vi "chaosui-crest-cu-setstate.vi"(5 "dev_state":T1=enum."init", 6 "timeout (10000)":i32=10000, 7 "cuname":string, 8 "handleConnection":T3) -> (0 "dev_error":bool, 1 "timestamp":u64, 2 "nok":i32, 3 "dev_state_out":T1, 4 "output out":string)   [LabVIEW 2014, in "chaosui-crest.lvlib"]
doc: "uint64_t chaos_crest_cu_get(chaos_crest_handle_t h,const char*cuname,char*output,int maxsize);"
uses:
  chaosui-crest.lvlib
  <vilib>/httpClient/ClientHandle.ctl
  ChaosDevState.ctl
  <vilib>/httpClient/LabVIEWHTTPClient.lvlib
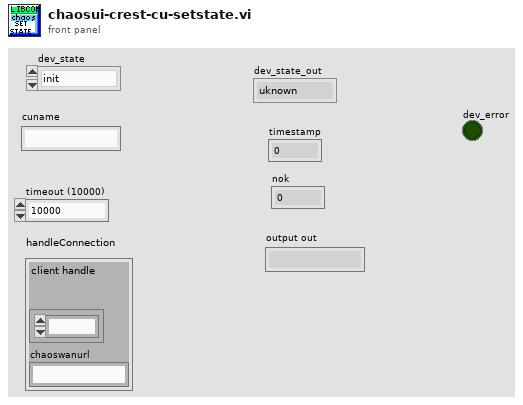
[diagram p1: front panel]
types:
  T1 = typedef "ChaosDevState.ctl" = enum16{"uknown", "stop", "init", "deinit", "start"}
  T2 = typedef "LabVIEWHTTPClient.lvlib/ClientHandle.ctl" = refnum<k1>
  T3 = cluster{"client handle":T2, "chaoswanurl":string}
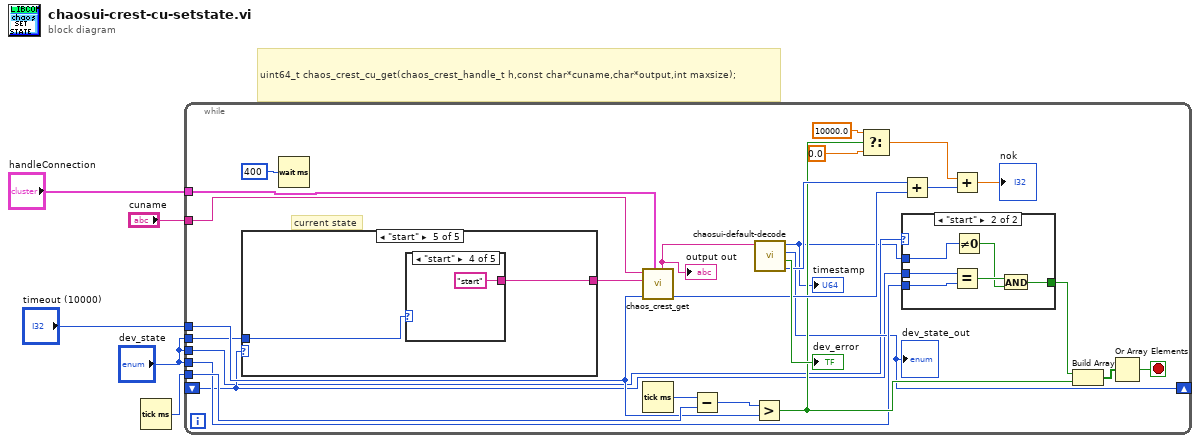
[diagram p0: block diagram]
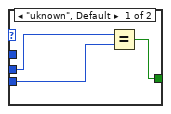
[diagram p2: hidden frame]
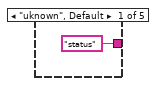
[diagram p3: hidden frame]
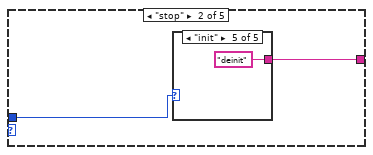
[diagram p4: hidden frame]
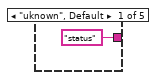
[diagram p5: hidden frame]
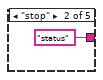
[diagram p6: hidden frame]
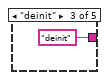
[diagram p7: hidden frame]
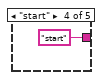
[diagram p8: hidden frame]
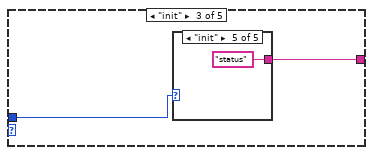
[diagram p9: hidden frame]
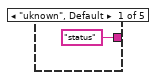
[diagram p10: hidden frame]
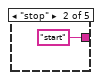
[diagram p11: hidden frame]
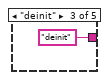
[diagram p12: hidden frame]
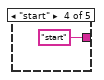
[diagram p13: hidden frame]
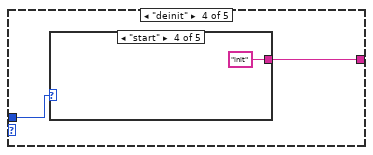
[diagram p14: hidden frame]
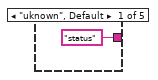
[diagram p15: hidden frame]
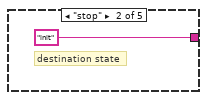
[diagram p16: hidden frame]
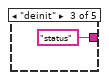
[diagram p17: hidden frame]
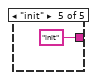
[diagram p18: hidden frame]
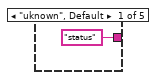
[diagram p19: hidden frame]
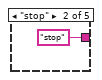
[diagram p20: hidden frame]
diagram:
  # "uint64_t chaos_crest_cu_get(chaos_crest_handle_t h,const char*cuname,char*output,int maxsize);"
  n1 = Tick Count (ms)() -> (millisecond timer value=w2:u32)
  n2 = while {
    tunnel: "handleConnection" -> [w30]
    tunnel: "timeout (10000)" -> [w21]
    tunnel: "cuname" -> [w29]
    tunnel: "dev_state" -> [w13]
    tunnel: w2 -> [w22]
    shift-right: [w11] -> _
    shift-left: _ -> [w10]
    tunnel: "dev_state" -> [w9]
    tunnel: "dev_state" -> [w8]
    stop <- w26 stop-if-true
    # "current state"
    n3 = case shown="\"start\"" w10 {
      tunnel: ["status" w43 w50 w57 w64] -> w12
      tunnel: w9 -> [_ w44 w51 w58 w65]
      frame "uknown", Default {
      }
      frame "stop" {
        n4 = case shown="\"init\"" w44 {
          tunnel: ["status" "status" "deinit" "start" "deinit"] -> w43
          frame "uknown", Default {
          }
          frame "stop" {
          }
          frame "deinit" {
          }
          frame "start" {
          }
          frame "init" {
          }
        }
      }
      frame "init" {
        n5 = case shown="\"init\"" w51 {
          tunnel: ["status" "start" "deinit" "start" "status"] -> w50
          frame "uknown", Default {
          }
          frame "stop" {
          }
          frame "deinit" {
          }
          frame "start" {
          }
          frame "init" {
          }
        }
      }
      frame "deinit" {
        n6 = case shown="\"start\"" w58 {
          tunnel: ["status" "init" "status" "init" "init"] -> w57
          frame "uknown", Default {
          }
          frame "stop" {
            # "destination state"
          }
          frame "deinit" {
          }
          frame "start" {
          }
          frame "init" {
          }
        }
      }
      frame "start" {
        n7 = case shown="\"start\"" w65 {
          tunnel: ["status" "stop" "stop" "start" "stop"] -> w64
          frame "uknown", Default {
          }
          frame "stop" {
          }
          frame "deinit" {
          }
          frame "start" {
          }
          frame "init" {
          }
        }
      }
    }
    n8 = Wait (ms)(milliseconds to wait=u32 400) -> ()  [unwired: 1 out]
    n9 = call "chaos_crest_get.vi"("cuname"=w29, "cmd"=w12, "timeout (10000)"=w21, "handleConnection"=w30) -> ("body"=w28:string, "nok"=w27:i32)  [unwired: 4 in, 1 out]
    "output out" <- w28
    n10 = Tick Count (ms)() -> (millisecond timer value=w23:u32)
    n11 = Subtract(x=w23, y=w22) -> (x-y=w20:u32)
    n12 = Greater?(x=w20, y=w21) -> (0:w17:bool)
    n13 = call "chaosui-default-decode.vi"("JSON string"=w28) -> ("parse_error"=w31:i32, "dev_error"=→"dev_error":bool, "dev_state"=w11:T1, "timestamp"=w7:u64)  [unwired: 3 in, 1 out]
    "timestamp" <- w7
    "dev_state_out" <- w11
    n14 = Select(t=10000.0, s=w17, f=0.0) -> (s? t:f=w14:dbl)
    n15 = Add(x=w31, y=w27) -> (x+y=w25:i32)
    n16 = case shown="\"start\"" w8 {
      tunnel: [w33 w36] -> w6
      tunnel: w13 -> [w34 w41]
      tunnel: w10 -> [w35 w40]
      tunnel: w7 -> [_ w39]
      frame "uknown", Default {
        n17 = Equal?(x=w35, y=w34) -> (x = y?=w33:bool)
      }
      frame "start" {
        n18 = Equal?(x=w40, y=w41) -> (x = y?=w38:bool)
        n19 = Not Equal To 0?(x=w39) -> (x != 0?=w37:bool)
        n20 = And(x=w38, y=w37) -> (x .and. y?=w36:bool)
      }
    }
    n21 = Add(x=w14, y=w25) -> (x+y=→"nok":dbl)
    n22 = Build Array(w6, w17) -> (w19:bool[])
    n23 = Or Array Elements(Boolean array=w19) -> (logical OR=w26:bool)
  }
